vi "Report_Type.vi"(8 "error in (no error)":errorcluster, 11 "IB_EXE in":refnum<class "IB_EXE.lvclass">) -> (0 "error out":errorcluster, 2 "type":string, 3 "IB_EXE out":refnum<class "IB_EXE.lvclass">)   [LabVIEW 2020, in "IB_EXE.lvclass"]
uses:
  <vilib>/AppBuilder/IB_Classes/Source/Container/Build/EXE/IB_EXE.lvclass
  <vilib>/AppBuilder/IB_Classes/Source/Container/Build/EXE/IB_EXE.lvclass/IB_EXE.ctl
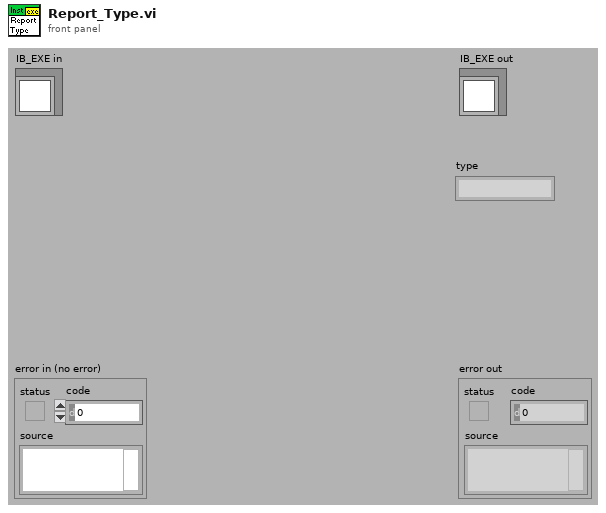
[diagram p1: front panel]
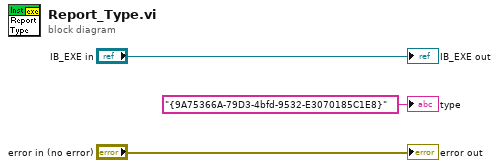
[diagram p0: block diagram]
diagram:
  "error out" <- "error in (no error)"
  "IB_EXE out" <- "IB_EXE in"
  "type" <- "{9A75366A-79D3-4bfd-9532-E3070185C1E8}" ("type")
